vi "P9374AEasilyUse_v5.vi"(0 "Resource String":string="PXI10::CHASSIS1::SLOT1::FUNC0::INSTR" caption="resource name", 1 "S-Parameter":u16(ring) items=["S11", "S12", "S21", "S22", "All"], 2 "Source Power (dBm)":dbl=-40.0 format="%#_13g", 3 "Start Frequency":dbl=300000.0 format="%#_13p", 4 "Stop Frequency":dbl=20000000000.0 format="%#_13p", 5 "error in":errorcluster, 6 "Source":u16(ring) items=["Both ports", "Port1", "Port2"], 9 "Averaging":bool, 10 "Path":path=path "P:/", 11 "Averaging Factor":i32=1, 12 "Filename":string="test", 13 "Avg Wait Time":u32=10000, 17 "Run":bool, 18 "Stop":bool) -> (14 "S Parameter":string="S21", 19 "error out":errorcluster)   [LabVIEW 2016]
uses:
  <userlib>/_OpenG.lib/error/error.llb/Filter Error Codes (Array)__ogtk.vi
  <instrlib>/Agilent NA/Agilent NA.lvlib
panel:
  in  "Notes":string
  out "Graph":dbl[](graph)
  in  "Channel":i32=1
  in  "Measurement":i32=1
  in  "Data Points":i32=2048 format="%.3g"
  # "Warning: Before running this VI, open the I/O interface first!!!!!!"
  # "Press \"Run!\" button to set the parameters and take data once. Press \"STOP!\" button to exit the VNA control."
  # "Settings"
  # "Data"
  # "Usually do not need to change."
  # "The S-parameters\nS11: Source1, Receiver1\nS12: Source2, Receiver1\nS21: Source1, Receiver2\nS22: Source2, Receiver2\nAll: Take all four data, save four files."
  # "If True"
  # "Set the maximun data points = the data points input."
  # "Other things need to be set from front panel:\nIF band width (always default 100kHz?)"
  # "About waiting time: Approximately, for 2048 data points, the averaging factor rate is 3 per second. \n                                    Eg. 2048 data points, averaging 30 times needs 10 second wait time."
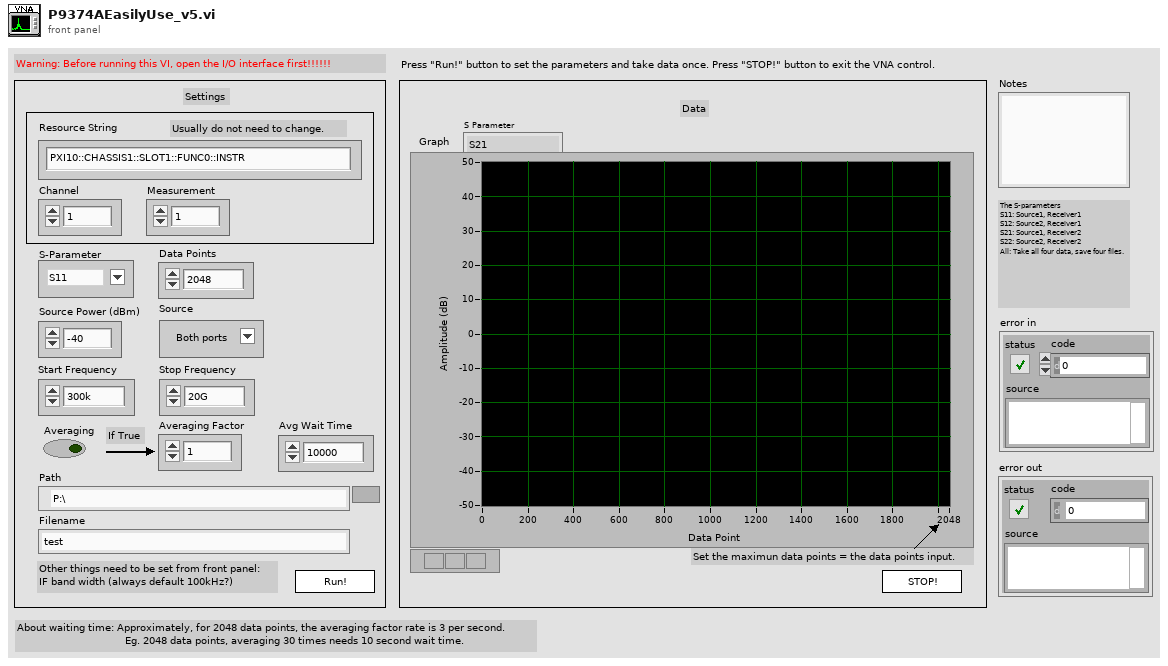
[diagram p1: front panel]
types:
  T1 = enum32{"invalid app kind", "Development System", "Run Time System", "Student Edition", "Embedded LabVIEW", "Evaluation", "Custom"}
  T2 = enum32{"Invalid", "Standard", "Closed", "Hidden", "Minimized", "Maximized"}
  T3 = cluster{"Core":cluster{"Current VI Reference":refnum<vi>, "Close Panel on Exit?":bool}, "Inst Handle":refnum<k15>, "Str C/M":cluster{"Measurement":string, "Channel":string}, "Data Pts":i32, "Graph":dbl[], "S-parameter":string, "Power":dbl, "Freq Range":cluster{"Start Freq":dbl, "Stop Freq":dbl}}
  T4 = cluster{"Current VI Reference":refnum<vi>, "Close Panel on Exit?":bool}
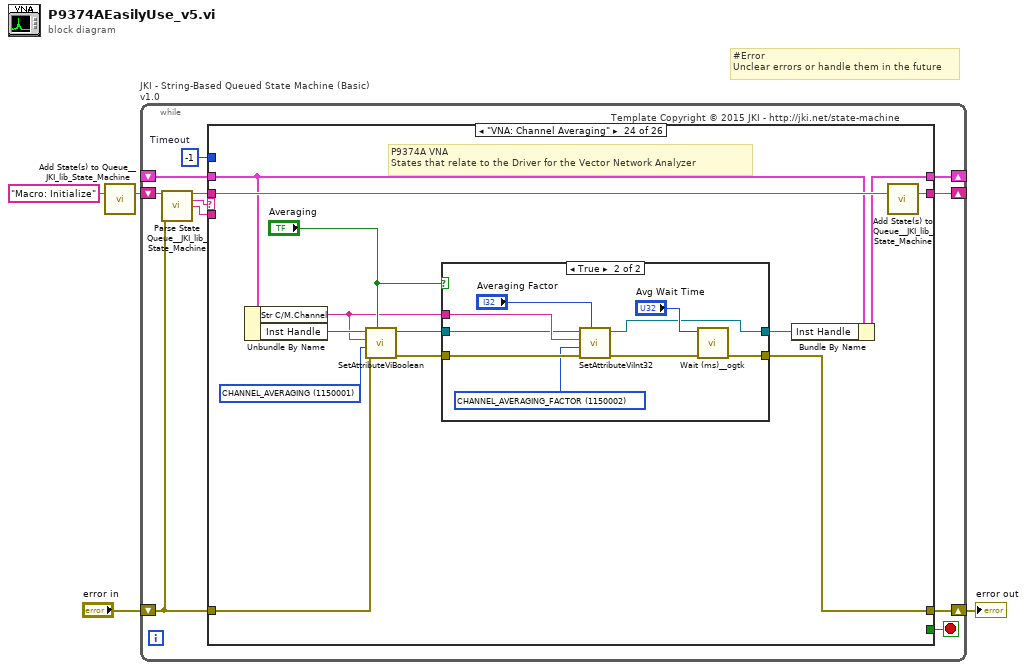
[diagram p0: block diagram]
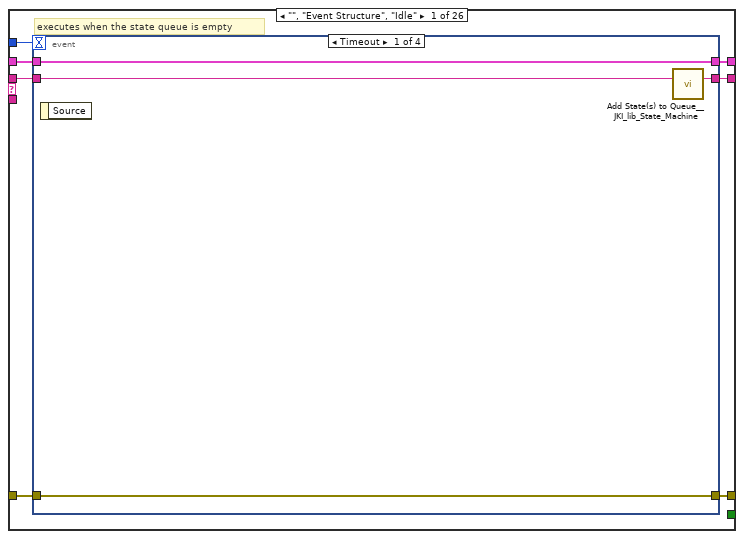
[diagram p2: hidden frame]
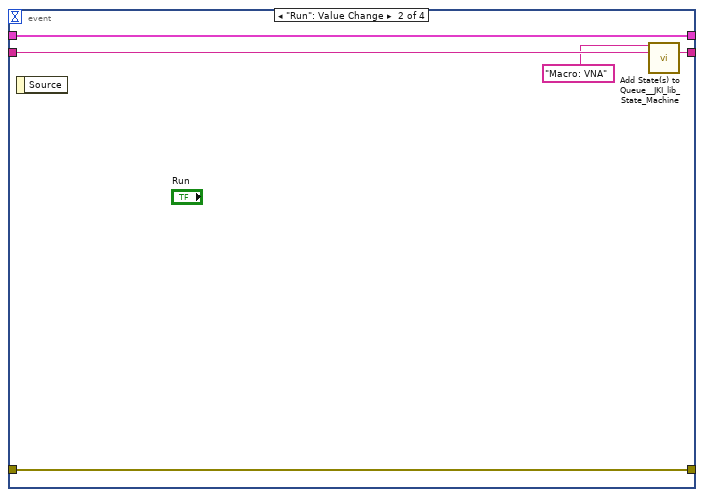
[diagram p3: hidden frame]
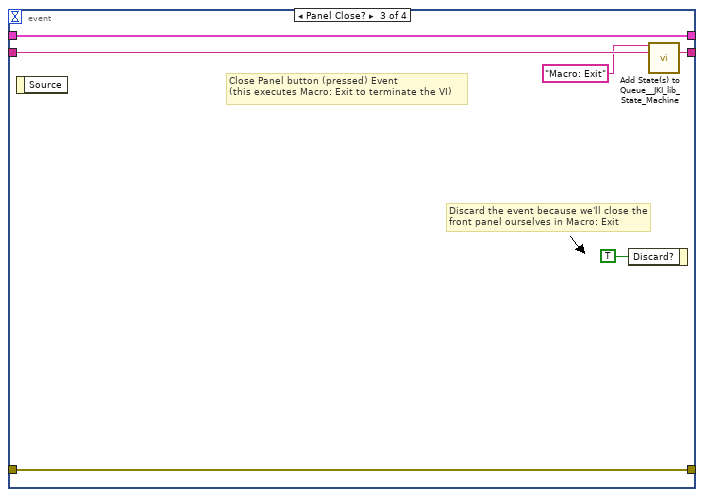
[diagram p4: hidden frame]
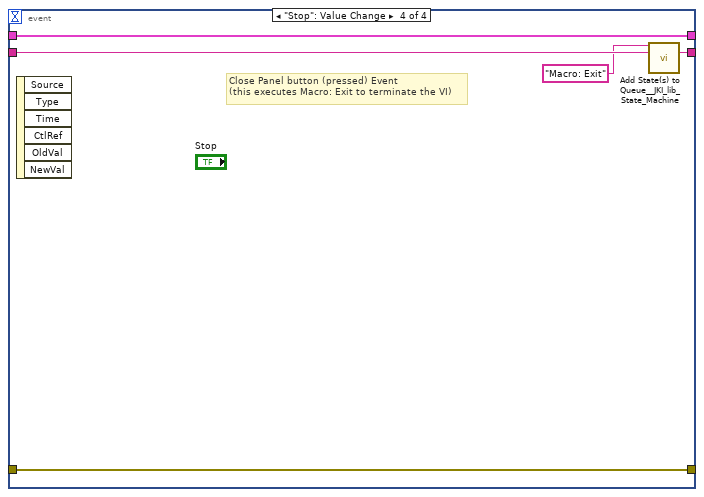
[diagram p5: hidden frame]
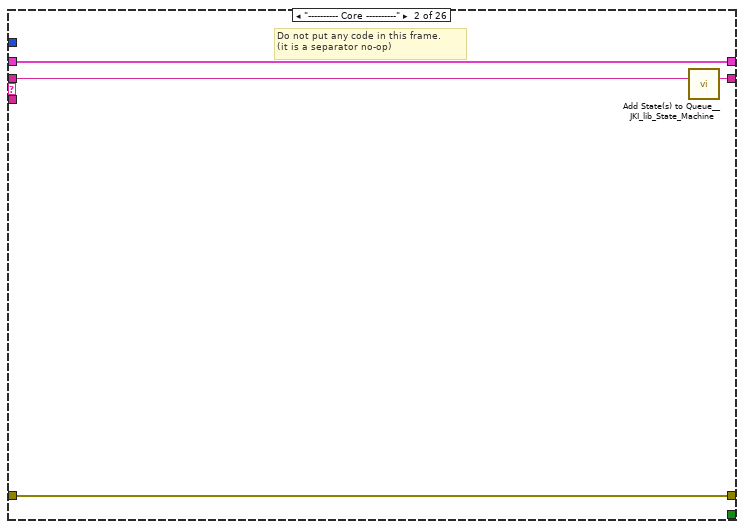
[diagram p6: hidden frame]
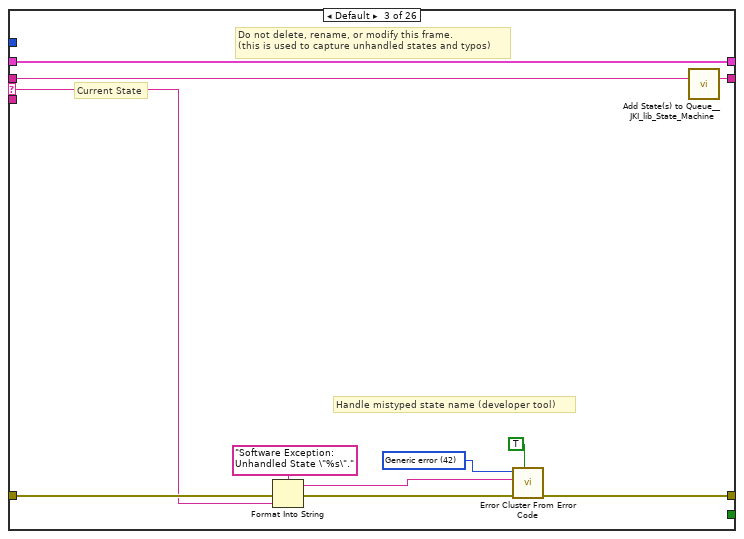
[diagram p7: hidden frame]
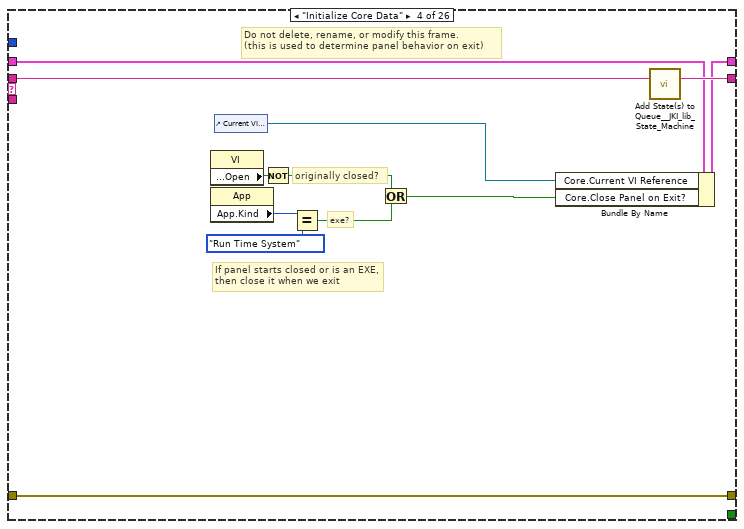
[diagram p8: hidden frame]
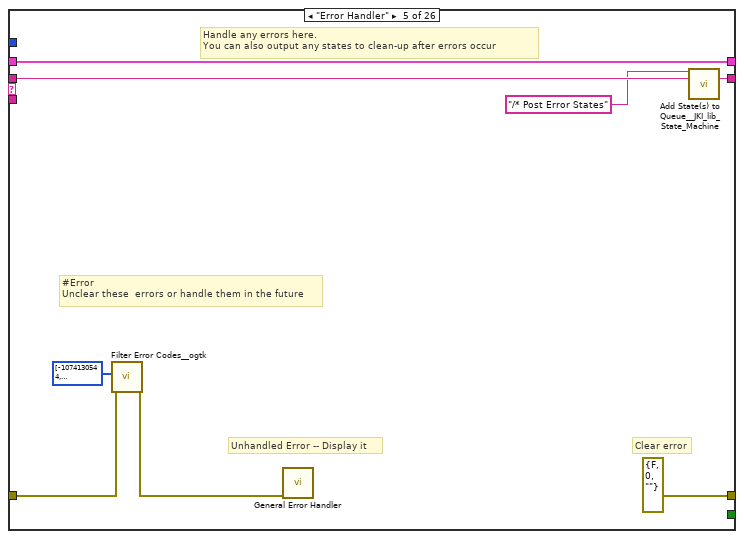
[diagram p9: hidden frame]
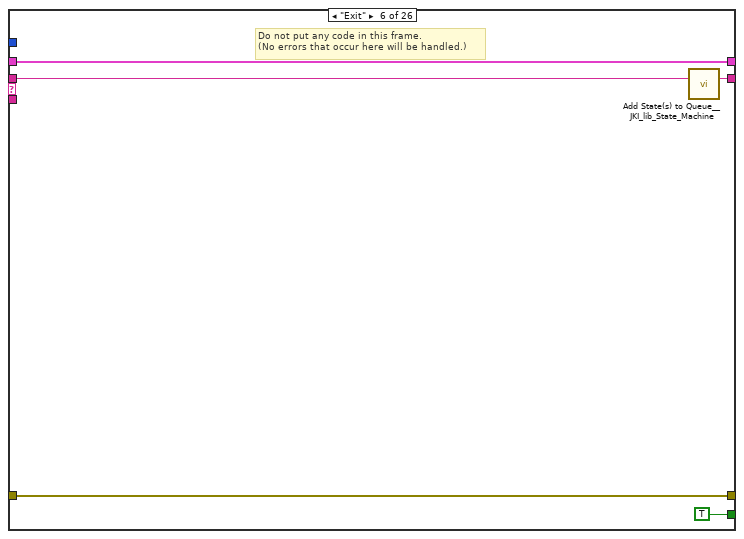
[diagram p10: hidden frame]
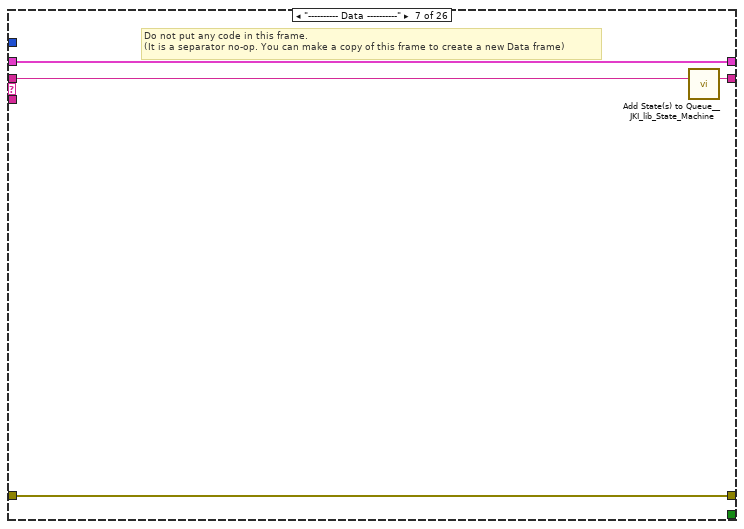
[diagram p11: hidden frame]
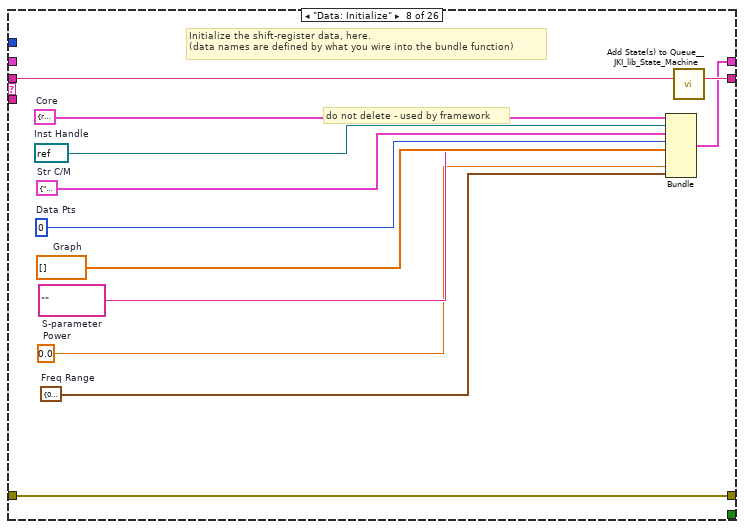
[diagram p12: hidden frame]
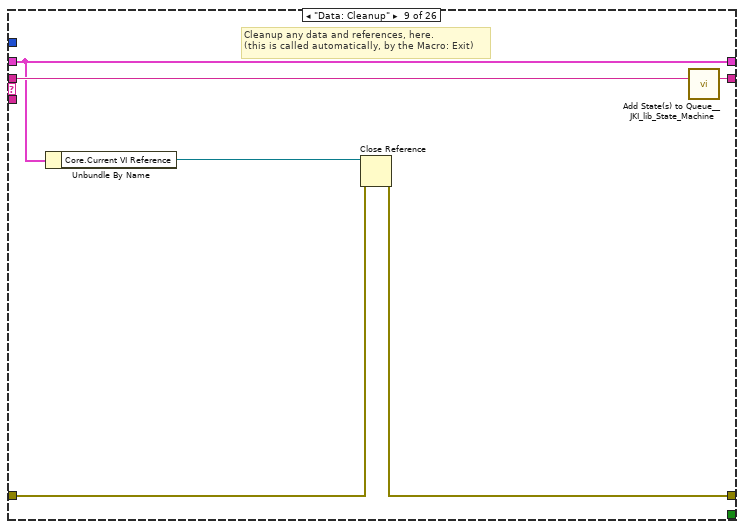
[diagram p13: hidden frame]
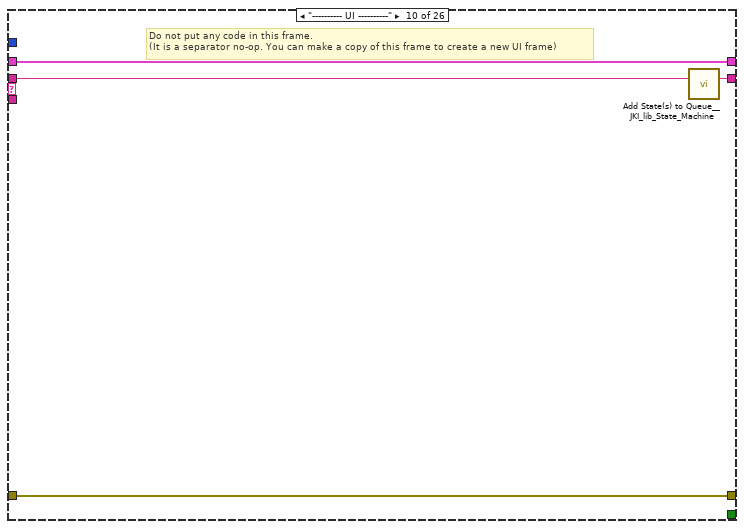
[diagram p14: hidden frame]
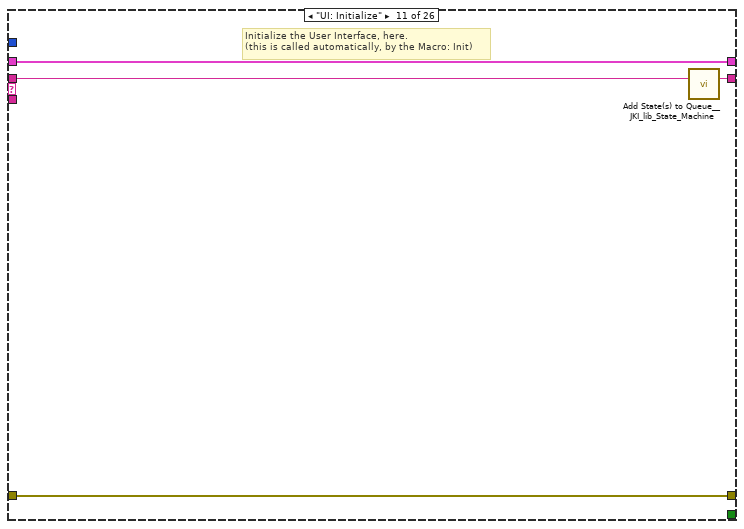
[diagram p15: hidden frame]
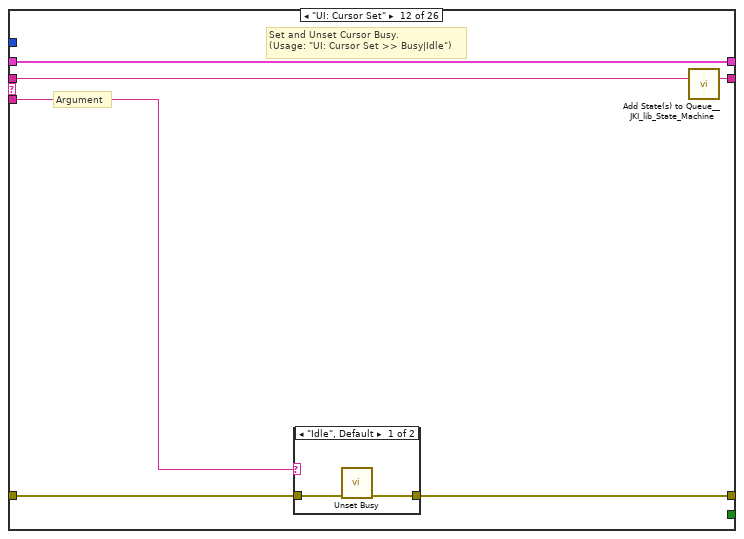
[diagram p16: hidden frame]
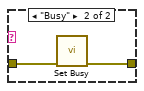
[diagram p17: hidden frame]
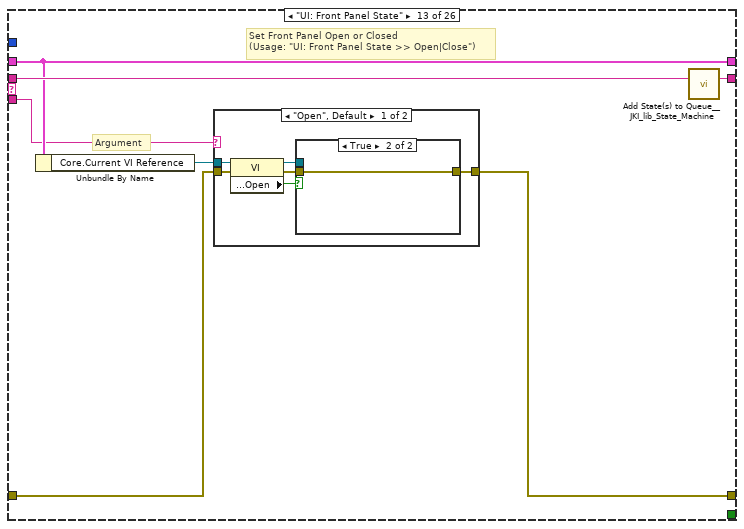
[diagram p18: hidden frame]
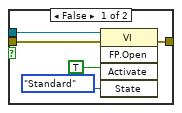
[diagram p19: hidden frame]
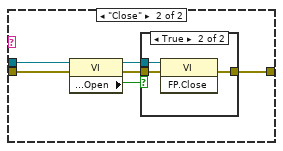
[diagram p20: hidden frame]
diagram:
  # "#Error\nUnclear errors or handle them in the future"
  n1 = call <vilib>:"Add State(s) to Queue__JKI_lib_State_Machine.vi"("State(s) in (\"\")"="Macro: Initialize") -> ("States Out"=w4:string)  [unwired: 14 in]
  n2 = while "JKI - String-Based Queued State Machine (Basic) v1.0" {
    shift-right: [w8] -> _
    shift-left: _ -> [w7]
    shift-right: [w11] -> w2
    shift-left: "error in" -> [w5]
    shift-right: [w10] -> _
    shift-left: w4 -> [w12]
    stop <- w9 stop-if-true
    w6 = -1  # Timeout
    # "Template Copyright © 2015 JKI - http://jki.net/state-machine"
    n3 = call <vilib>:"Parse State Queue__JKI_lib_State_Machine.vi"("State Queue"=w12, "Error In (no error)"=w5) -> ("Remaining States"=w14:string, "Current State"=w15:string, "Arguments"=w13:string)  [unwired: 11 in]
    n4 = case shown="\"VNA: Channel Averaging\"" w15 {
      selector: w15 -> [_ _ w47 _ _ _ _ _ _ _ _ _ _ _ _ _ _ _ _ _ _ _ _ _ _ _]
      tunnel: w14 -> [w22 w46 w51 w69 w77 w82 w86 w98 w104 w108 w112 w118 w129 w155 w160 w169 w215 w219 w235 w247 w282 w293 w312 w333 w358 w383]
      tunnel: w13 -> [_ _ _ _ _ _ _ _ _ _ _ w113 w123 _ _ _ _ _ _ _ _ _ w301 _ _ _]
      tunnel: w7 -> [w20 w43 w49 w60 w74 w80 w83 _ w99 w105 w110 w116 w125 w152 w157 w166 w212 w216 w233 w242 w280 w291 w304 w328 w353 w381]
      tunnel: [w19 w44 w53 w66 errorcluster {"status"=FALSE, "code"=0, "source"=""} ("error out") w79 w84 w95 w100 w106 w109 w114 w126 w153 w158 w167 w213 w217 w222 w244 w274 w284 w300 w330 w350 w369] -> w11
      tunnel: w5 -> [w18 w44 w52 w66 w71 w79 w84 w95 w101 w106 w109 w115 w127 w153 w158 w167 w213 w217 w223 w245 w275 w285 w299 w323 w351 w369]
      tunnel: [w21 w45 w50 w68 w76 w81 w85 w97 w103 w107 w111 w117 w128 w154 w159 w168 w214 w218 w234 w246 w281 w292 w311 w332 w357 w382] -> w10
      tunnel: [_ _ _ _ _ TRUE _ _ _ _ _ _ _ _ _ _ _ _ _ _ _ _ _ _ _ _] -> w9
      tunnel: [w17 w43 w49 w67 w74 w80 w83 w96 w99 w105 w110 w116 w125 w152 w157 w166 w212 w216 w232 w241 w279 w290 w303 w331 w352 w381] -> w8
      tunnel: w6 -> [w16 _ _ _ _ _ _ _ _ _ _ _ _ _ _ _ _ _ _ _ _ _ _ _ _ _]
      frame "", "Event Structure", "Idle" {
        # "executes when the state queue is empty"
        n5 = event shown="[0] Timeout" {
          selector: _ -> [_ _ _ _]
          dyn-events: _ -> [_ _ _ _]
          timeout: w16 -> [_ _ _ _]
          tunnel: w22 -> [w26 w31 w37 w42]
          tunnel: [w25 w30 w36 w41] -> w21
          tunnel: w20 -> [w23 w28 w34 w39]
          tunnel: [w24 w29 w35 w40] -> w19
          tunnel: w18 -> [w24 w29 w35 w40]
          tunnel: [w23 w28 w34 w39] -> w17
          event Timeout {
            n6 = event-data() -> ()  [unwired: 1 in, 1 out]
            n7 = call <vilib>:"Add State(s) to Queue__JKI_lib_State_Machine.vi"("State(s) in (\"\")"=w26) -> ("States Out"=w25:string)  [unwired: 14 in]
          }
          event "Run": Value Change {
            n8 = event-data() -> ()  [unwired: 1 in, 1 out]
            n9 = call <vilib>:"Add State(s) to Queue__JKI_lib_State_Machine.vi"("State(s) in Front (\"\")"="Macro: VNA", "State(s) in (\"\")"=w31) -> ("States Out"=w30:string)  [unwired: 13 in]
          }
          event Panel Close? {
            # "Discard the event because we'll close the front panel ourselves in Macro: Exit"
            # "Close Panel button (pressed) Event\n(this executes Macro: Exit to terminate the VI)"
            n10 = event-data() -> ()  [unwired: 1 in, 1 out]
            n11 = event-data("Discard?"=TRUE) -> ()  [unwired: 1 in, 1 out]
            n12 = call <vilib>:"Add State(s) to Queue__JKI_lib_State_Machine.vi"("State(s) in Front (\"\")"="Macro: Exit", "State(s) in (\"\")"=w37) -> ("States Out"=w36:string)  [unwired: 13 in]
          }
          event "Stop": Value Change {
            # "Close Panel button (pressed) Event\n(this executes Macro: Exit to terminate the VI)"
            n13 = event-data() -> ()  [unwired: 1 in, 6 out]
            n14 = call <vilib>:"Add State(s) to Queue__JKI_lib_State_Machine.vi"("State(s) in Front (\"\")"="Macro: Exit", "State(s) in (\"\")"=w42) -> ("States Out"=w41:string)  [unwired: 13 in]
          }
        }
      }
      frame "---------- Core ----------" {
        # "Do not put any code in this frame.\n(it is a separator no-op)"
        n15 = call <vilib>:"Add State(s) to Queue__JKI_lib_State_Machine.vi"("State(s) in (\"\")"=w46) -> ("States Out"=w45:string)  [unwired: 14 in]
      }
      frame Default {
        w56 = 42 items=["No error", "Argument error", "Memory is full", "Out of zone", "End of file", "File already open", "Generic file I/O error", "File not found", "File permission error", "Disk is full", "Duplicate path", "Too many files open", "System feature not enabled", "Resource file not found", "Cannot add resource", "Resource not found", "Image not found", "Image memory error", "Pen does not exist", "Config type invalid", "Config token not found", "Config parse error", "Config memory error", "Bad external code format", "Bad external code offset", "External code not present", "Null window", "Destroy window error", "Null menu", "Print aborted", "Bad print record", "Print driver error", "Windows error during printing", "Memory error during printing", "Print dialog error", "Generic print error", "Invalid device refnum", "Device not found", "Device parameter error", "Device unit error", "Cannot open device", "Device call aborted", "Generic error", "Cancelled by user", "Object ID too low", "Object ID too high", "Object not in heap", "Unknown heap", "Unknown object (invalid DefProc)", "Unknown object (DefProc not in table)", "Message out of range", "Invalid (null) method", "Unknown message", "Manager call not supported", "Bad address", "Network operation in progress", "Network operation timed out", "Connection is busy", "Network attribute not supported", "Network error", "Address in use", "System out of memory", "Connection aborted", "Connection refused", "Not connected", "Already connected", "Connection closed", "Initialization error (interapplication manager)", "Bad occurrence", "Wait on unbound occurrence handler", "Occurrence queue overflow", "Datalog type conflict", "Unused", "Unrecognized type (interapplication manager)", "Memory corrupt", "Failed to make temporary DLL", "Old CIN version", "Drag socket not found", "Failed to load drop-object", "Failed to register OLE object", "Failed to release OLE object", "Format specifier type mismatch", "Unknown format specifier", "Too few format specifiers", "Too many format specifiers", "Scan failed", "Newer CIN version", "Error converting to variant", "Runtime menu error", "Password tampered", "Variant attribute not found", "Incompatible variant data type", "Event data is not available", "Event Store is not present", "Occurrence is not found", "Event Queue is not created", "Event info is not available", "Refnum passed is NULL", "Error retrieving Class GUID", "Error retrieving CoClass GUID", "Error retrieving TypeLib GUID.", "Bad built application magic bytes.", "Specific driver is different from the specific driver associated with the Logical Name.", "There is no session opened to the class driver.", "Max Error", "MAX - Error with config objects", "MAX - Error loading configuration", "MAX - Group not supported"]
        # "Current State"
        # "Do not delete, rename, or modify this frame.\n(this is used to capture unhandled states and typos)"
        # "Handle mistyped state name (developer tool)"
        n16 = Format Into String(format string="Software Exception: Unhandled State \"%s\"." ("message"), error in=w52, w47) -> (resulting string=w55:string, error out=w54:errorcluster)  [unwired: 1 in]
        n17 = call <vilib>:"Error Cluster From Error Code.vi"("show call chain? (False)"=TRUE, "error in (no error)"=w54, "error message (\"\")"=w55, "error code (0)"=w56) -> ("error out"=w53:errorcluster)  [unwired: 5 in]
        n18 = call <vilib>:"Add State(s) to Queue__JKI_lib_State_Machine.vi"("State(s) in (\"\")"=w51) -> ("States Out"=w50:string)  [unwired: 14 in]
      }
      frame "Initialize Core Data" {
        # "Do not delete, rename, or modify this frame.\n(this is used to determine panel behavior on exit)"
        # "originally closed?"
        # "exe?"
        # "If panel starts closed or is an EXE, then close it when we exit"
        n19 = property class="VI"() -> ("Front Panel.Open"=w65:bool)  [unwired: 2 in, 2 out]
        n20 = property class="App"() -> ("App.Kind"=w64:T1)  [unwired: 2 in, 2 out]
        n21 = control-ref of="Current VI Reference"() -> (w58:refnum<vi>)
        n22 = Not(x=w65) -> (.not. x?=w62:bool)
        n23 = Equal?(x=w64, y=T1."Run Time System" ("Application:Kind")) -> (x = y?=w61:bool)
        n24 = Or(x=w62, y=w61) -> (x .or. y?=w59:bool)
        n25 = Bundle By Name(cluster=w60, "Core.Current VI Reference"=w58, "Core.Close Panel on Exit?"=w59) -> (w67:T3)
        n26 = call <vilib>:"Add State(s) to Queue__JKI_lib_State_Machine.vi"("State(s) in (\"\")"=w69) -> ("States Out"=w68:string)  [unwired: 14 in]
      }
      frame "Error Handler" {
        # "#Error\nUnclear these  errors or handle them in the future"
        # "Unhandled Error -- Display it"
        # "Handle any errors here.\nYou can also output any states to clean-up after errors occur"
        # "Clear error"
        n27 = call-poly <userlib>:"Filter Error Codes__ogtk.vi"("Error In"=w71, "Error Codes to Filter"=i32[] [-1074130544, -1074134944]) -> ("Error Out"=w70:errorcluster)  [unwired: 7 in, 2 out]
        n28 = call <vilib>:"General Error Handler.vi"("error in (no error)"=w70) -> ()  [unwired: 10 in, 5 out]
        n29 = call <vilib>:"Add State(s) to Queue__JKI_lib_State_Machine.vi"("State(s) in Front (\"\")"="/* Post Error States", "State(s) in (\"\")"=w77) -> ("States Out"=w76:string)  [unwired: 13 in]
      }
      frame "Exit" {
        # "Do not put any code in this frame.\n(No errors that occur here will be handled.)"
        n30 = call <vilib>:"Add State(s) to Queue__JKI_lib_State_Machine.vi"("State(s) in (\"\")"=w82) -> ("States Out"=w81:string)  [unwired: 14 in]
      }
      frame "---------- Data ----------" {
        # "Do not put any code in this frame.\n(It is a separator no-op. You can make a copy of this frame to create a new Data frame)"
        n31 = call <vilib>:"Add State(s) to Queue__JKI_lib_State_Machine.vi"("State(s) in (\"\")"=w86) -> ("States Out"=w85:string)  [unwired: 14 in]
      }
      frame "Data: Initialize" {
        w87 = cluster{"Start Freq":dbl, "Stop Freq":dbl} {"Start Freq"=0.0, "Stop Freq"=0.0}  # Freq Range
        w88 = 0.0  # Power
        w89 = ""  # S-parameter
        w90 = dbl[] []  # Graph
        w91 = 0  # Data Pts
        w92 = cluster{"Measurement":string, "Channel":string} {"Measurement"="Measurement1", "Channel"="Channel1"}  # Str C/M
        w93 = refnum<k15> "PXI10::CHASSIS1::SLOT1::FUNC0::INSTR (94)"  # Inst Handle
        w94 = T4 {"Current VI Reference"=refnum, "Close Panel on Exit?"=FALSE}  # Core
        # "do not delete - used by framework"
        # "Initialize the shift-register data, here.\n(data names are defined by what you wire into the bundle function)"
        n32 = Bundle("Core"=w94, "Inst Handle"=w93, "Str C/M"=w92, "Data Pts"=w91, "Graph"=w90, "S-parameter"=w89, "Power"=w88, "Freq Range"=w87) -> (w96:T3)  [unwired: 1 in]
        n33 = call <vilib>:"Add State(s) to Queue__JKI_lib_State_Machine.vi"("State(s) in (\"\")"=w98) -> ("States Out"=w97:string)  [unwired: 14 in]
      }
      frame "Data: Cleanup" {
        # "Cleanup any data and references, here.\n(this is called automatically, by the Macro: Exit)"
        n34 = Unbundle By Name(w99) -> ("Core.Current VI Reference"=w102:refnum<vi>)
        n35 = Close Reference(reference=w102, error in (no error)=w101) -> (error out=w100:errorcluster)
        n36 = call <vilib>:"Add State(s) to Queue__JKI_lib_State_Machine.vi"("State(s) in (\"\")"=w104) -> ("States Out"=w103:string)  [unwired: 14 in]
      }
      frame "---------- UI ----------" {
        # "Do not put any code in this frame.\n(It is a separator no-op. You can make a copy of this frame to create a new UI frame)"
        n37 = call <vilib>:"Add State(s) to Queue__JKI_lib_State_Machine.vi"("State(s) in (\"\")"=w108) -> ("States Out"=w107:string)  [unwired: 14 in]
      }
      frame "UI: Initialize" {
        # "Initialize the User Interface, here.\n(this is called automatically, by the Macro: Init)"
        n38 = call <vilib>:"Add State(s) to Queue__JKI_lib_State_Machine.vi"("State(s) in (\"\")"=w112) -> ("States Out"=w111:string)  [unwired: 14 in]
      }
      frame "UI: Cursor Set" {
        # "Argument"
        # "Set and Unset Cursor Busy.\n(Usage: \"UI: Cursor Set >> Busy|Idle\")"
        n39 = case shown="\"Idle\", Default" w113 {
          tunnel: w115 -> [w120 w122]
          tunnel: [w119 w121] -> w114
          frame "Idle", Default {
            n40 = call <vilib>:"Unset Busy.vi"("error in (no error)"=w120) -> ("error out"=w119:errorcluster)  [unwired: 10 in]
          }
          frame "Busy" {
            n41 = call <vilib>:"Set Busy.vi"("error in (no error)"=w122) -> ("error out"=w121:errorcluster)  [unwired: 9 in, 1 out]
          }
        }
        n42 = call <vilib>:"Add State(s) to Queue__JKI_lib_State_Machine.vi"("State(s) in (\"\")"=w118) -> ("States Out"=w117:string)  [unwired: 14 in]
      }
      frame "UI: Front Panel State" {
        # "Argument"
        # "Set Front Panel Open or Closed\n(Usage: \"UI: Front Panel State >> Open|Close\")"
        n43 = Unbundle By Name(w125) -> ("Core.Current VI Reference"=w124:refnum<vi>)
        n44 = case shown="\"Open\", Default" w123 {
          tunnel: w127 -> [w133 w146]
          tunnel: [w135 w147] -> w126
          tunnel: w124 -> [w134 w144]
          frame "Open", Default {
            n45 = property class="VI"(reference=w134, error in=w133) -> (reference out=w131:refnum<vi>, error out=w132:errorcluster, "Front Panel.Open"=w130:bool)
            n46 = case shown="True" w130 {
              tunnel: [w138 w141] -> w135
              tunnel: w132 -> [w137 w141]
              tunnel: w131 -> [w136 _]
              frame False {
                n47 = invoke class="VI" method="FP.Open"(reference=w136, error in=w137, "Activate"=TRUE, "State"=T2."Standard") -> (error out=w138:errorcluster)  [unwired: 1 in, 4 out]
              }
              frame True {
              }
            }
          }
          frame "Close" {
            n48 = property class="VI"(reference=w144, error in=w146) -> (reference out=w143:refnum<vi>, error out=w145:errorcluster, "Front Panel.Open"=w142:bool)
            n49 = case shown="True" w142 {
              tunnel: [w148 w151] -> w147
              tunnel: w145 -> [w148 w150]
              tunnel: w143 -> [_ w149]
              frame False {
              }
              frame True {
                n50 = invoke class="VI" method="FP.Close"(reference=w149, error in=w150) -> (error out=w151:errorcluster)  [unwired: 1 in, 2 out]
              }
            }
          }
        }
        n51 = call <vilib>:"Add State(s) to Queue__JKI_lib_State_Machine.vi"("State(s) in (\"\")"=w129) -> ("States Out"=w128:string)  [unwired: 14 in]
      }
      frame "---------- Macro ----------" {
        # "Do not put any code in this frame.\n(It is a separator no-op. You can make a copy of this frame to create a new Macro frame)"
        n52 = call <vilib>:"Add State(s) to Queue__JKI_lib_State_Machine.vi"("State(s) in (\"\")"=w155) -> ("States Out"=w154:string)  [unwired: 14 in]
      }
      frame "Macro: Initialize" {
        w156 = "Data: Initialize\nInitialize Core Data\nUI: Initialize\nUI: Front Panel State >> Open"  # Data: Initialize Initialize Core Data UI: Initialize UI: Front Panel State >> Open
        # "Initialization Macro\n(This is called once, when the VI starts)"
        n53 = call <vilib>:"Add State(s) to Queue__JKI_lib_State_Machine.vi"("State(s) in Front (\"\")"=w156, "State(s) in (\"\")"=w160) -> ("States Out"=w159:string)  [unwired: 13 in]
      }
      frame "Macro: VNA" {
        # "Do not put any code in this frame.\n(It is a separator no-op. You can make a copy of this frame to create a new Macro frame)"
        n54 = case shown="4" "S-Parameter" {
          tunnel: "VNA: Init\nVNA: Set Power\nVNA: Set Freq\nVNA: Set Data Pts" -> [w173 w179 w185 w191 w198]
          tunnel: "VNA: Channel Averaging\nVNA: DAQ\nVNA: Save" -> [w171 w177 w184 w190 w196]
          tunnel: [w170 w178 w183 w189 w194] -> w162
          tunnel: "VNA: Set S Param" -> [w172 w176 w182 w188 w197]
          frame 0, Default {
            n55 = call <vilib>:"Build State String with Arguments__JKI_lib_State_Machine.vi"("Arguments (\"\")"="S11", "State"=w172) -> ("State with Arguments"=w174:string)  [unwired: 4 in]
            n56 = call <vilib>:"Add State(s) to Queue__JKI_lib_State_Machine.vi"("State(s) in Front (\"\")"=w173, "State(s) in (\"\")"=w174, "State(s) at Back (\"\")"=w171) -> ("States Out"=w170:string)  [unwired: 12 in]
          }
          frame 1 {
            n57 = call <vilib>:"Build State String with Arguments__JKI_lib_State_Machine.vi"("Arguments (\"\")"="S12", "State"=w176) -> ("State with Arguments"=w180:string)  [unwired: 4 in]
            n58 = call <vilib>:"Add State(s) to Queue__JKI_lib_State_Machine.vi"("State(s) in Front (\"\")"=w179, "State(s) in (\"\")"=w180, "State(s) at Back (\"\")"=w177) -> ("States Out"=w178:string)  [unwired: 12 in]
          }
          frame 2 {
            n59 = call <vilib>:"Build State String with Arguments__JKI_lib_State_Machine.vi"("Arguments (\"\")"="S21", "State"=w182) -> ("State with Arguments"=w186:string)  [unwired: 4 in]
            n60 = call <vilib>:"Add State(s) to Queue__JKI_lib_State_Machine.vi"("State(s) in Front (\"\")"=w185, "State(s) in (\"\")"=w186, "State(s) at Back (\"\")"=w184) -> ("States Out"=w183:string)  [unwired: 12 in]
          }
          frame 3 {
            n61 = call <vilib>:"Build State String with Arguments__JKI_lib_State_Machine.vi"("Arguments (\"\")"="S22", "State"=w188) -> ("State with Arguments"=w192:string)  [unwired: 4 in]
            n62 = call <vilib>:"Add State(s) to Queue__JKI_lib_State_Machine.vi"("State(s) in Front (\"\")"=w191, "State(s) in (\"\")"=w192, "State(s) at Back (\"\")"=w190) -> ("States Out"=w189:string)  [unwired: 12 in]
          }
          frame 4 {
            n63 = for {
              shift-right: [w204] -> w194
              shift-left: w198 -> [w205]
              tunnel: string[] ["S11", "S12", "S21", "S22"] -> [w202] mode=indexing
              tunnel: w197 -> [w200]
              tunnel: w196 -> [w199]
              n64 = call <vilib>:"Build State String with Arguments__JKI_lib_State_Machine.vi"("Arguments (\"\")"=w202, "State"=w200) -> ("State with Arguments"=w203:string)  [unwired: 4 in]
              n65 = call <vilib>:"Add State(s) to Queue__JKI_lib_State_Machine.vi"("State(s) in (\"\")"=w203, "State(s) at Back (\"\")"=w199) -> ("States Out"=w201:string)  [unwired: 13 in]
              n66 = call <vilib>:"Add State(s) to Queue__JKI_lib_State_Machine.vi"("State(s) in (\"\")"=w205, "State(s) at Back (\"\")"=w201) -> ("States Out"=w204:string)  [unwired: 13 in]
            }
          }
        }
        n67 = call <vilib>:"Add State(s) to Queue__JKI_lib_State_Machine.vi"("State(s) in Front (\"\")"=w162, "State(s) in (\"\")"=w169) -> ("States Out"=w168:string)  [unwired: 13 in]
      }
      frame "Macro: Exit" {
        # "Exit Macro\n(This is called once, when the VI exits)"
        n68 = Unbundle By Name(w212) -> ("Core.Close Panel on Exit?"=w211:bool)
        n69 = Select(t="UI: Front Panel State >> Close", s=w211, f="") -> (s? t:f=w208:string)
        n70 = call <vilib>:"Add State(s) to Queue__JKI_lib_State_Machine.vi"("State(s) in (\"\")"=w208, "State(s) at Back (\"\")"="Data: Cleanup\nExit") -> ("States Out"=w206:string)  [unwired: 13 in]
        n71 = call <vilib>:"Add State(s) to Queue__JKI_lib_State_Machine.vi"("State(s) in Front (\"\")"=w206, "State(s) in (\"\")"=w215) -> ("States Out"=w214:string)  [unwired: 13 in]
      }
      frame "---------- VNA ----------" {
        # "P9374A VNA\nStates that relate to the Driver for the Vector Network Analyzer"
        n72 = call <vilib>:"Add State(s) to Queue__JKI_lib_State_Machine.vi"("State(s) in (\"\")"=w219) -> ("States Out"=w218:string)  [unwired: 14 in]
      }
      frame "VNA: Init" {
        n73 = call <instrlib>:"Initialize With Options.vi"("error in (no error)"=w223, "resource string"="Resource String") -> ("error out"=w222:errorcluster, "instrument handle out"=w221:refnum<k15>)  [unwired: 8 in]
        n74 = Number To Decimal String(number="Channel") -> (decimal integer string=w229:string)  [unwired: 1 in]
        n75 = Number To Decimal String(number="Measurement") -> (decimal integer string=w230:string)  [unwired: 1 in]
        n76 = Concatenate Strings("Channel" ("string"), w229) -> (w228:string)
        n77 = Concatenate Strings("Measurement" ("string"), w230) -> (w227:string)
        n78 = Bundle By Name(cluster=w233, "Inst Handle"=w221, "Str C/M.Channel"=w228, "Str C/M.Measurement"=w227) -> (w232:T3)
        n79 = call <vilib>:"Add State(s) to Queue__JKI_lib_State_Machine.vi"("State(s) in (\"\")"=w235) -> ("States Out"=w234:string)  [unwired: 14 in]
      }
      frame "VNA: Set Power" {
        n80 = Unbundle By Name(w242) -> ("Inst Handle"=w243:refnum<k15>, "Str C/M.Channel"=w237:string)
        n81 = case shown="0, Default" "Source" {
          tunnel: w245 -> [w256 w259 w266]
          tunnel: [w248 w258 w265] -> w244
          tunnel: w243 -> [w257 w262 w269]
          tunnel: [w254 w264 w271] -> w240
          tunnel: "Source Power (dBm)" -> [w253 w263 w270]
          tunnel: w237 -> [w251 w261 w268]
          tunnel: [w253 w263 w270] -> w236
          frame 0, Default {
            w255 = 1 ("PortVal")
            n82 = call <instrlib>:"Channel Source Power Set Level.vi"("Val"=w253, "error in (no error)"=w256, "PortVal"=w255, "instrument handle"=w257) -> ("error out"=w249:errorcluster, "instrument handle out"=w252:refnum<k15>)  [unwired: 6 in]
            n83 = Increment(x=w255) -> (x+1=w250:i32)
            n84 = call <instrlib>:"Channel Source Power Set Level.vi"("Val"=w253, "error in (no error)"=w249, "PortVal"=w250, "RepCapIdentifier"=w251, "instrument handle"=w252) -> ("error out"=w248:errorcluster, "instrument handle out"=w254:refnum<k15>)  [unwired: 5 in]
          }
          frame 1 {
            n85 = call <instrlib>:"Channel Source Power Set Level.vi"("Val"=w263, "error in (no error)"=w259, "PortVal"=1, "RepCapIdentifier"=w261, "instrument handle"=w262) -> ("error out"=w258:errorcluster, "instrument handle out"=w264:refnum<k15>)  [unwired: 5 in]
          }
          frame 2 {
            n86 = call <instrlib>:"Channel Source Power Set Level.vi"("Val"=w270, "error in (no error)"=w266, "PortVal"=2, "RepCapIdentifier"=w268, "instrument handle"=w269) -> ("error out"=w265:errorcluster, "instrument handle out"=w271:refnum<k15>)  [unwired: 5 in]
          }
        }
        n87 = Bundle By Name(cluster=w242, "Inst Handle"=w240, "Power"=w236) -> (w241:T3)
        n88 = call <vilib>:"Add State(s) to Queue__JKI_lib_State_Machine.vi"("State(s) in (\"\")"=w247) -> ("States Out"=w246:string)  [unwired: 14 in]
      }
      frame "VNA: Set Freq" {
        # "P9374A VNA\nStates that relate to the Driver for the Vector Network Analyzer"
        n89 = Unbundle By Name(w280) -> ("Inst Handle"=w277:refnum<k15>, "Str C/M.Channel"=w276:string)
        n90 = call <instrlib>:"Channel Stimulus Range Configure Start Stop.vi"("StopVal"="Stop Frequency", "error in (no error)"=w275, "StartVal"="Start Frequency", "RepCapIdentifier"=w276, "instrument handle"=w277) -> ("error out"=w274:errorcluster, "instrument handle out"=w273:refnum<k15>)  [unwired: 5 in]
        n91 = Bundle By Name(cluster=w280, "Inst Handle"=w273, "Freq Range.Start Freq"="Start Frequency", "Freq Range.Stop Freq"="Stop Frequency") -> (w279:T3)
        n92 = call <vilib>:"Add State(s) to Queue__JKI_lib_State_Machine.vi"("State(s) in (\"\")"=w282) -> ("States Out"=w281:string)  [unwired: 14 in]
      }
      frame "VNA: Set Data Pts" {
        w286 = u32 1150007 items=["CHANNEL_AVERAGING_FACTOR"=1150002, "CHANNEL_MEASUREMENT_ELECTRICAL_DELAY_MEDIUM"=1150178, "CHANNEL_MEASUREMENT_ELECTRICAL_DELAY_UNITS"=1150175, "CHANNEL_MEASUREMENT_FORMAT"=1150014, "CHANNEL_MEASUREMENT_LIMIT_NUMBER"=1150020, "CHANNEL_MEASUREMENT_TIME_DOMAIN_GATING_SHAPE"=1150140, "CHANNEL_MEASUREMENT_TIME_DOMAIN_GATING_TYPE"=1150144, "CHANNEL_MEASUREMENT_TIME_DOMAIN_PARAMETERS"=1150137, "CHANNEL_MEASUREMENT_TIME_DOMAIN_TRANSFORM_MODE"=1150147, "CHANNEL_MEASUREMENT_TRACE_MATH"=1150017, "CHANNEL_POINTS"=1150007, "CHANNEL_SWEEP_MODE"=1150009, "CHANNEL_SWEEP_TYPE"=1150012, "CHANNEL_TRIGGER_MODE"=1150013, "DISPLAY_ARRANGE_WINDOWS"=1150181, "SYSTEM_TIME_OUT_MILLISECONDS"=1150040, "TRIGGER_SOURCE"=1150042, "WINDOW_SIZE"=1150133, "WINDOW_TABLE"=1150134] ("AttributeID")
        # "P9374A VNA\nStates that relate to the Driver for the Vector Network Analyzer"
        n93 = Unbundle By Name(w291) -> ("Inst Handle"=w288:refnum<k15>, "Str C/M.Channel"=w287:string)
        n94 = call <instrlib>:"SetAttributeViInt32.vi"("AttributeValue"="Data Points", "error in (no error)"=w285, "AttributeID"=w286, "RepCapIdentifier"=w287, "instrument handle"=w288) -> ("error out"=w284:errorcluster, "instrument handle out"=w289:refnum<k15>)  [unwired: 5 in]
        n95 = Bundle By Name(cluster=w291, "Data Pts"="Data Points", "Inst Handle"=w289) -> (w290:T3)
        n96 = call <vilib>:"Add State(s) to Queue__JKI_lib_State_Machine.vi"("State(s) in (\"\")"=w293) -> ("States Out"=w292:string)  [unwired: 14 in]
      }
      frame "VNA: Set S Param" {
        # "P9374A VNA\nStates that relate to the Driver for the Vector Network Analyzer"
        n97 = Unbundle By Name(w304) -> ("Inst Handle"=w296:refnum<k15>, "Str C/M.Channel"=w307:string, "Str C/M.Measurement"=w306:string)
        n98 = case shown="\"S22\"" w301 {
          tunnel: [w314 w316 w318 w320] -> w297
          tunnel: [w313 w315 w317 w319] -> w294
          frame "S11", Default {
            w313 = 1  # Receiver Port
            w314 = 1  # Source Port
          }
          frame "S21" {
            w315 = 2  # Receiver Port
            w316 = 1  # Source Port
          }
          frame "S12" {
            w317 = 1  # Receiver Port
            w318 = 2  # Source Port
          }
          frame "S22" {
            w319 = 2  # Receiver Port
            w320 = 2  # Source Port
          }
        }
        n99 = Concatenate Strings(w307, ":" ("string"), w306) -> (w295:string)
        n100 = Number To Decimal String(number=w294) -> (decimal integer string=w309:string)  [unwired: 1 in]
        n101 = Number To Decimal String(number=w297) -> (decimal integer string=w308:string)  [unwired: 1 in]
        n102 = call <instrlib>:"Channel Measurement Set S Parameter.vi"("NewSourcePortVal"=w297, "error in (no error)"=w299, "NewReceiverPortVal"=w294, "RepCapIdentifier"=w295, "instrument handle"=w296) -> ("error out"=w300:errorcluster, "instrument handle out"=w298:refnum<k15>)  [unwired: 5 in]
        n103 = Concatenate Strings("S" ("string"), w309, w308) -> (w302:string)
        "S Parameter" <- w302
        n104 = Bundle By Name(cluster=w304, "S-parameter"=w302, "Inst Handle"=w298) -> (w303:T3)
        n105 = call <vilib>:"Add State(s) to Queue__JKI_lib_State_Machine.vi"("State(s) in (\"\")"=w312) -> ("States Out"=w311:string)  [unwired: 14 in]
      }
      frame "VNA: Channel Averaging" {
        w324 = u32 1150001 items=["CHANNEL_AVERAGING"=1150001, "CHANNEL_CORRECTION"=1150003, "CHANNEL_MEASUREMENT_LIMIT_ENABLE"=1150018, "CHANNEL_MEASUREMENT_MARKER_ENABLED"=1150022, "CHANNEL_MEASUREMENT_MARKER_MARKER_TRACK_ENABLED"=1150023, "CHANNEL_MEASUREMENT_SMOOTHING"=1150015, "CHANNEL_MEASUREMENT_TIME_DOMAIN_COUPLING_STATE"=1150136, "CHANNEL_MEASUREMENT_TIME_DOMAIN_GATING_ENABLE"=1150139, "CHANNEL_MEASUREMENT_TIME_DOMAIN_TRANSFORM_ENABLE"=1150146, "CHANNEL_MEASUREMENT_TRACE_ENABLE_TRACE_MAX"=1150182, "CHANNEL_PORT_EXTENSION_STATUS"=1150008, "CHANNEL_SOURCEPOWER_COUPLING"=1150031, "CHANNEL_SWEEP_TIME_AUTO"=1150011, "DISPLAY_ENABLED"=1150036, "GUIDED_CALIBRATION_ADVANCED_E_CAL_AUTO_ORIENTATION"=1150116, "SIMULATE"=1050005, "SYSTEM_POWER_ENABLED"=1150184, "SYSTEM_TRACE_ENABLED"=1150041, "WINDOW_STATE"=1150183, "WINDOW_TITLE_STATE"=1150132] ("AttributeID")
        # "P9374A VNA\nStates that relate to the Driver for the Vector Network Analyzer"
        n106 = Unbundle By Name(w328) -> ("Str C/M.Channel"=w325:string, "Inst Handle"=w326:refnum<k15>)
        n107 = call <instrlib>:"SetAttributeViBoolean.vi"("AttributeValue (Off)"="Averaging", "error in (no error)"=w323, "AttributeID"=w324, "RepCapIdentifier"=w325, "instrument handle"=w326) -> ("error out"=w322:errorcluster, "instrument handle out"=w321:refnum<k15>)  [unwired: 5 in]
        n108 = case shown="True" "Averaging" {
          tunnel: w322 -> [w335 w341]
          tunnel: [w335 w344] -> w330
          tunnel: w321 -> [w334 w338]
          tunnel: [w334 w337] -> w329
          tunnel: w325 -> [_ w339]
          frame False {
          }
          frame True {
            w340 = u32 1150002 items=["CHANNEL_AVERAGING_FACTOR"=1150002, "CHANNEL_MEASUREMENT_ELECTRICAL_DELAY_MEDIUM"=1150178, "CHANNEL_MEASUREMENT_ELECTRICAL_DELAY_UNITS"=1150175, "CHANNEL_MEASUREMENT_FORMAT"=1150014, "CHANNEL_MEASUREMENT_LIMIT_NUMBER"=1150020, "CHANNEL_MEASUREMENT_TIME_DOMAIN_GATING_SHAPE"=1150140, "CHANNEL_MEASUREMENT_TIME_DOMAIN_GATING_TYPE"=1150144, "CHANNEL_MEASUREMENT_TIME_DOMAIN_PARAMETERS"=1150137, "CHANNEL_MEASUREMENT_TIME_DOMAIN_TRANSFORM_MODE"=1150147, "CHANNEL_MEASUREMENT_TRACE_MATH"=1150017, "CHANNEL_POINTS"=1150007, "CHANNEL_SWEEP_MODE"=1150009, "CHANNEL_SWEEP_TYPE"=1150012, "CHANNEL_TRIGGER_MODE"=1150013, "DISPLAY_ARRANGE_WINDOWS"=1150181, "SYSTEM_TIME_OUT_MILLISECONDS"=1150040, "TRIGGER_SOURCE"=1150042, "WINDOW_SIZE"=1150133, "WINDOW_TABLE"=1150134] ("AttributeID")
            n109 = call <instrlib>:"SetAttributeViInt32.vi"("AttributeValue"="Averaging Factor", "error in (no error)"=w341, "AttributeID"=w340, "RepCapIdentifier"=w339, "instrument handle"=w338) -> ("error out"=w342:errorcluster, "instrument handle out"=w337:refnum<k15>)  [unwired: 5 in]
            n110 = call <userlib>:"Wait (ms)__ogtk.vi"("error in (no error)"=w342, "milliseconds to wait"="Avg Wait Time") -> ("error out"=w344:errorcluster)  [unwired: 8 in, 1 out]
          }
        }
        n111 = Bundle By Name(cluster=w328, "Inst Handle"=w329) -> (w331:T3)
        n112 = call <vilib>:"Add State(s) to Queue__JKI_lib_State_Machine.vi"("State(s) in (\"\")"=w333) -> ("States Out"=w332:string)  [unwired: 14 in]
      }
      frame "VNA: DAQ" {
        # "P9374A VNA\nStates that relate to the Driver for the Vector Network Analyzer"
        n113 = Unbundle By Name(w353) -> ("Inst Handle"=w347:refnum<k15>, "Str C/M.Channel"=w355:string, "Str C/M.Measurement"=w354:string, "Data Pts"=w345:i32)
        n114 = Concatenate Strings(w355, ":", w354) -> (w346:string)
        n115 = call <instrlib>:"Channel Measurement Fetch Formatted.vi"("error in (no error)"=w351, "RetValBufferSize"=w345, "RepCapIdentifier"=w346, "instrument handle"=w347) -> ("error out"=w350:errorcluster, "RetVal"=w348:dbl[], "instrument handle out"=w349:refnum<k15>)  [unwired: 4 in, 1 out]
        "Graph" <- w348
        n116 = Bundle By Name(cluster=w353, "Inst Handle"=w349, "Graph"=w348) -> (w352:T3)
        n117 = call <vilib>:"Add State(s) to Queue__JKI_lib_State_Machine.vi"("State(s) in (\"\")"=w358) -> ("States Out"=w357:string)  [unwired: 14 in]
      }
      frame "VNA: Save" {
        w372 = "_" ("string")
        n118 = Unbundle By Name(w381) -> ("Power"=w375:dbl, "S-parameter"=w379:string, "Graph"=w368:dbl[], "Freq Range.Start Freq"=w362:dbl, "Freq Range.Stop Freq"=w363:dbl, "Data Pts"=w359:i32)
        n119 = Greater Than 0?(x=w375) -> (x > 0?=w377:bool)
        n120 = case shown="False" w377 {
          tunnel: ["n" "p"] -> w376
          frame False {
          }
          frame True {
          }
        }
        n121 = Absolute Value(x=w375) -> (abs(x)=w374:dbl)
        n122 = Number To Decimal String(number=w374) -> (decimal integer string=w373:string)  [unwired: 1 in]
        n123 = Format Into String(format string="%.0p%s%.0p", w362, w372, w363) -> (resulting string=w370:string)  [unwired: 2 in, 1 out]
        n124 = for {
          N: w359 -> [_]
          tunnel: w363 -> [w392]
          tunnel: w362 -> [w390]
          tunnel: w359 -> [w386]
          tunnel: [w388] -> w361 mode=indexing
          i -> [w393]
          n125 = Subtract(x=w392, y=w390) -> (x-y=w387:dbl)
          n126 = Subtract(x=w386, y=1) -> (x-y=w384:i32)
          n127 = Divide(x=w387, y=w384) -> (x/y=w391:dbl)
          n128 = Multiply(x=w391, y=w393) -> (x*y=w389:dbl)
          n129 = Add(x=w390, y=w389) -> (x+y=w388:dbl)
        }
        n130 = Concatenate Strings("Filename", w372, w376, w373, "dBm" ("string"), w372, w370, w372, w379) -> (w365:string)
        n131 = Build Cluster Array(w361, w368) -> (w367:cluster{"Graph":dbl[]}[])
        n132 = call <vilib>:"LV to ITX AutoPlot.vi"("filename"=w365, "path"="Path", "Notes"="Notes", "Data"=w367, "wavenames (.Vx, etc)"=string[] ["Freq", "Amp"]) -> ()  [unwired: 10 in, 1 out]
        n133 = call <vilib>:"Add State(s) to Queue__JKI_lib_State_Machine.vi"("State(s) in (\"\")"=w383) -> ("States Out"=w382:string)  [unwired: 14 in]
      }
    }
  }
  "error out" <- w2
